vi "Check Link Validity in Sysdef.vi"(8 "error in (no error)":errorcluster, 10 "SysDef Root":refnum<k24>, 11 "Link":T2) -> (0 "error out":errorcluster, 3 "LinkData":T1)   [LabVIEW 2011]
uses:
  NationalInstruments.VeriStand.SystemStorage
  Controls/ECUMC Item.ctl
  Controls/LinkData.ctl
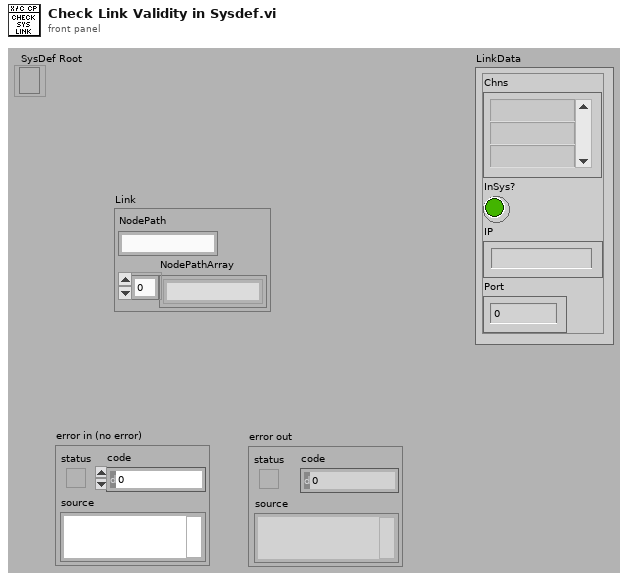
[diagram p1: front panel]
types:
  T1 = typedef "LinkData.ctl" = cluster{"Chns":string[], "InSys?":bool, "IP":string, "Port":u16}
  T2 = typedef "ECUMC Item.ctl" = cluster{"NodePath":string, "NodePathArray":string[]}
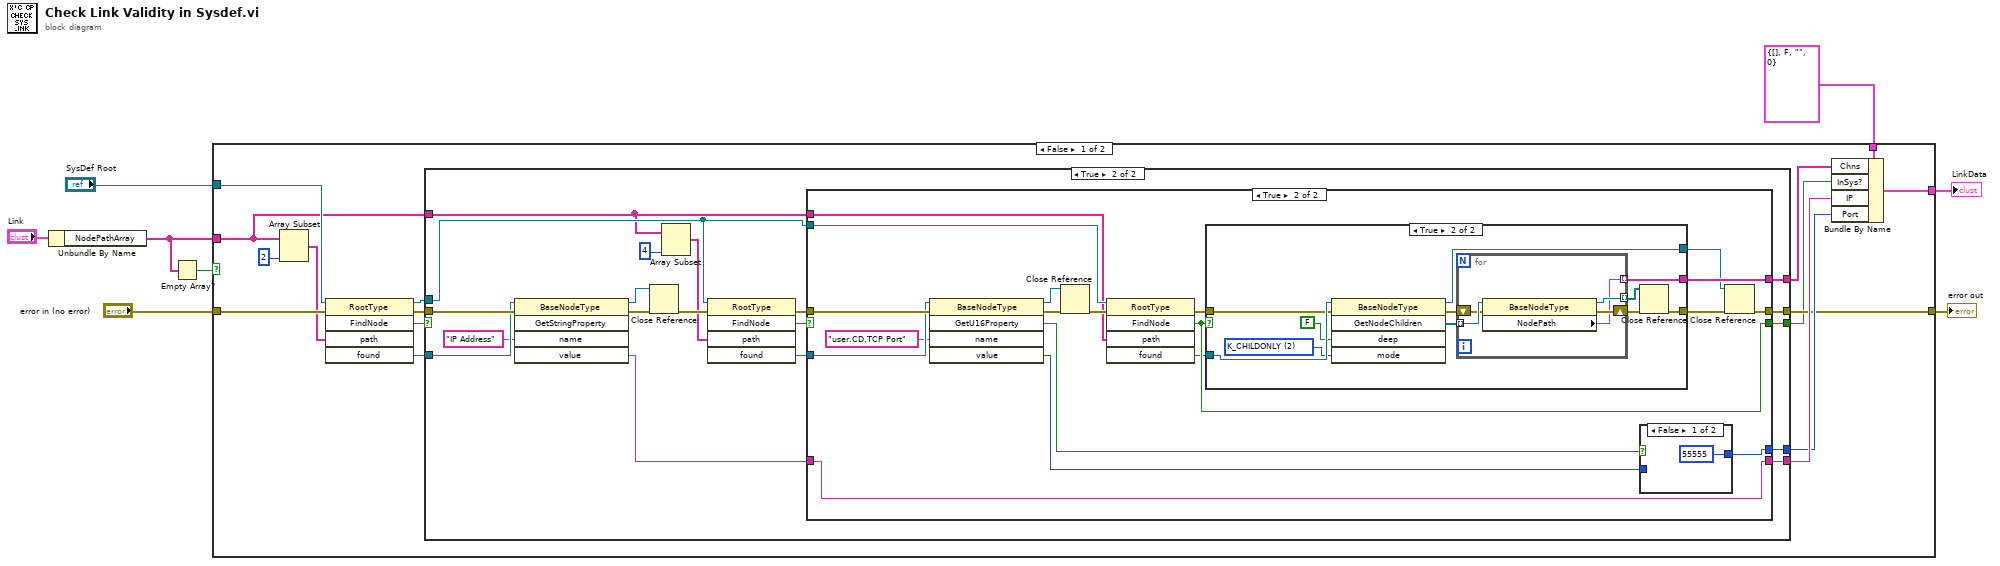
[diagram p0: block diagram]
diagram:
  n1 = Unbundle By Name("Link") -> ("NodePathArray"=w2:string[])
  n2 = Empty Array?(array=w2) -> (empty?=w1:bool)
  n3 = case shown="False" w1 {
    tunnel: "error in (no error)" -> [w24 w88]
    tunnel: [w16 w88] -> w7
    tunnel: "SysDef Root" -> [w12 _]
    tunnel: w2 -> [w11 _]
    tunnel: T1 {"Chns"=[], "InSys?"=FALSE, "IP"="", "Port"=0} ("LinkData") -> [w10 w89]
    tunnel: [w9 w89] -> w3
    frame False {
      n4 = Array Subset(array=w11, length=2) -> (w22:string[])  [unwired: 1 in]
      n5 = invoke class="RootType" method="FindNode"(reference=w12, error in=w24, "path"=w22) -> (reference out=w18:refnum<k24>, error out=w21:errorcluster, "FindNode"=w15:bool, "found"=w20:refnum<k24>)  [unwired: 2 in, 1 out]
      n6 = case shown="True" w15 {
        selector: w15 -> [w25 _]
        tunnel: w21 -> [w26 w45]
        tunnel: w20 -> [_ w44]
        tunnel: [_ w33] -> w19
        tunnel: w18 -> [_ w34]
        tunnel: [_ w40] -> w17
        tunnel: [w26 w39] -> w16
        tunnel: [w25 w28] -> w14
        tunnel: w11 -> [_ w31]
        tunnel: [_ w27] -> w13
        frame False {
        }
        frame True {
          n7 = invoke class="BaseNodeType" method="GetStringProperty"(reference=w44, error in=w45, "name"="IP Address") -> (reference out=w36:refnum<k24>, error out=w37:errorcluster, "value"=w32:string)  [unwired: 2 in, 2 out]
          n8 = Close Reference(reference=w36, error in (no error)=w37) -> (error out=w43:errorcluster)
          n9 = Array Subset(array=w31, length=4) -> (w29:string[])  [unwired: 1 in]
          n10 = invoke class="RootType" method="FindNode"(reference=w34, error in=w43, "path"=w29) -> (error out=w42:errorcluster, "FindNode"=w38:bool, "found"=w41:refnum<k24>)  [unwired: 2 in, 2 out]
          n11 = case shown="True" w38 {
            selector: w38 -> [w46 _]
            tunnel: w42 -> [w48 w67]
            tunnel: w41 -> [_ w66]
            tunnel: [_ w58] -> w40
            tunnel: [w48 w50] -> w39
            tunnel: w31 -> [_ w56]
            tunnel: w34 -> [_ w59]
            tunnel: [w47 w57] -> w33
            tunnel: w32 -> [w47 w57]
            tunnel: [w46 w55] -> w28
            tunnel: [_ w52] -> w27
            frame False {
            }
            frame True {
              n12 = invoke class="BaseNodeType" method="GetU16Property"(reference=w66, error in=w67, "name"="user.CD.TCP Port") -> (reference out=w63:refnum<k24>, error out=w62:errorcluster, "GetU16Property"=w65:bool, "value"=w64:u16)  [unwired: 2 in, 1 out]
              n13 = Close Reference(reference=w63, error in (no error)=w62) -> (error out=w60:errorcluster)
              n14 = invoke class="RootType" method="FindNode"(reference=w59, error in=w60, "path"=w56) -> (error out=w53:errorcluster, "FindNode"=w55:bool, "found"=w54:refnum<k24>)  [unwired: 2 in, 2 out]
              n15 = case shown="True" w55 {
                tunnel: w54 -> [w68 w80]
                tunnel: w53 -> [w69 w79]
                tunnel: [w69 w73] -> w51
                tunnel: [_ w72] -> w52
                tunnel: [w68 w70] -> w49
                frame False {
                }
                frame True {
                  w78 = 2 items=["K_BFS", "K_DFS", "K_CHILDONLY", "K_UP"] ("mode")
                  n16 = invoke class="BaseNodeType" method="GetNodeChildren"(reference=w80, error in=w79, "deep"=FALSE, "mode"=w78) -> (reference out=w70:refnum<k24>, error out=w71:errorcluster, "GetNodeChildren"=w76:refnum<k24>[])  [unwired: 1 in, 2 out]
                  n17 = for {
                    shift-right: [w83] -> w75
                    shift-left: w71 -> [w84]
                    tunnel: w76 -> [w85] mode=indexing
                    tunnel: [w82] -> w74 mode=indexing
                    tunnel: [w81] -> w72 mode=indexing
                    n18 = property class="BaseNodeType"(reference=w85, error in=w84) -> (reference out=w82:refnum<k24>, error out=w83:errorcluster, "NodePath"=w81:string)
                  }
                  n19 = Close Reference(reference=w74, error in (no error)=w75) -> (error out=w73:errorcluster)
                }
              }
              n20 = case shown="False" w65 {
                tunnel: [u16 55555 ("value") w87] -> w58
                tunnel: w64 -> [_ w87]
                frame False {
                }
                frame True {
                }
              }
              n21 = Close Reference(reference=w49, error in (no error)=w51) -> (error out=w50:errorcluster)
            }
          }
        }
      }
      n22 = Bundle By Name(cluster=w10, "Chns"=w13, "InSys?"=w14, "IP"=w19, "Port"=w17) -> (w9:T1)
    }
    frame True {
    }
  }
  "error out" <- w7
  "LinkData" <- w3
